vi "Status.Set.vi"(8 "error in (no error)":errorcluster, 9 "success?":bool, 10 "Data":u8[](array[numeric]), 11 "Status Ref":refnum<data-value>) -> (0 "error out":errorcluster)   [LabVIEW 2015, in "Diagnostics Addon Engine.lvlib"]
uses:
  Diagnostics Addon Engine.lvlib
  <vilib>/NI/NIVS Inline Async API/_Data Access Engine/Access Type Classes/Write/Write.lvclass
  <vilib>/NI/NIVS Inline Async API/_Data Access Engine/Access Type Classes/Write/Write.lvclass/Write.ctl
  <vilib>/NI/NIVS Inline Async API/_Data Access Engine/Data Access Engine/Methods/Write.Data.vi
  <vilib>/NI/NIVS Inline Async API/_Data Access Engine/Access Type Classes/Write/Write.ProcessData.vi
  <vilib>/NI/NIVS Inline Async API/_Data Access Engine/Data Access Engine/Data Access Engine.lvclass
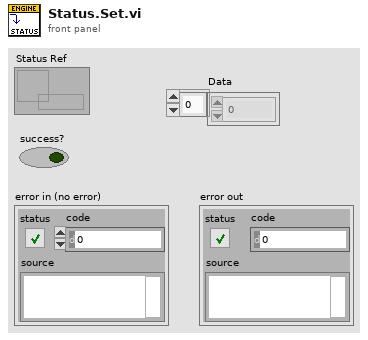
[diagram p1: front panel]
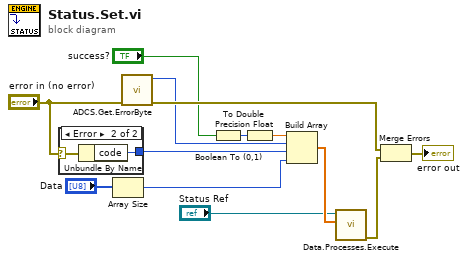
[diagram p0: block diagram]
diagram:
  n1 = case shown="Error" "error in (no error)" {
    selector: "error in (no error)" -> [_ w15]
    tunnel: [_ w14] -> w5
    frame No Error {
    }
    frame Error {
      n2 = Unbundle By Name(w15) -> ("code"=w14:i32)
    }
  }
  n3 = Array Size(array="Data") -> (size(s)=w4:i32)
  n4 = call "ADCS.Get.ErrorByte.vi"("error"="error in (no error)") -> ("error  out"=w13:errorcluster, "Error Byte"=w6:u8)  [unwired: 9 in]
  n5 = Boolean To (0,1)(Boolean="success?") -> (0, 1=w8:i16)
  n6 = To Double Precision Float(number=w8) -> (double precision float=w9:dbl)
  n7 = Build Array(w9, w6, w5, w4) -> (w3:dbl[])
  n8 = call-poly <vilib>:"Data.Processes.Execute.vi"("Values"=w3, "Ref"="Status Ref") -> ("error out"=w2:errorcluster)  [unwired: 9 in]
  n9 = Merge Errors(w13, w2) -> (→"error out":errorcluster)
